vi "Abort-lasing.vi"(8 "error in (no error)":errorcluster, 11 "Object ref in":T1) -> (0 "error out":errorcluster, 3 "Object ref out":T1)   [LabVIEW 2013, in "SLMControl.lvlib" / "SC-Main.lvclass"]
uses:
  SC-Main.lvclass
  Object-reference.ctl
  UI/Control-names.ctl
  Vision-actions.ctl
  SC-Main.lvclass/SC-Main.ctl
  Read Lasing control.vi
  Read UI.vi
  UI/Set-control-boolean.vi
  UI/Set-control-string.vi
  SM1000/SM1000.lvclass
  UI/SC-UI.lvclass
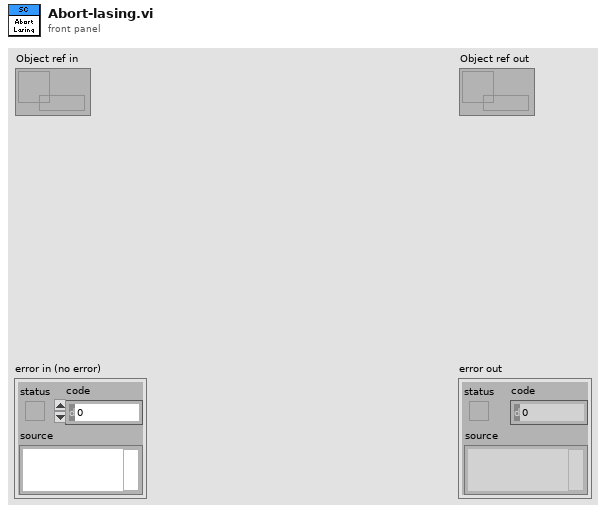
[diagram p1: front panel]
types:
  T1 = typedef "SLMControl.lvlib/SC-Main.lvclass/Object-reference.ctl" = refnum<data-value>
  T2 = typedef "SLMControl.lvlib/SC-Main.lvclass/Vision-actions.ctl" = enum16{"Activate", "Start", "Repeat", "Stop", "Exit"}
  T3 = typedef "SLMControl.lvlib/SC-UI.lvclass/Control-names.ctl" = enum16{"Com-in", "Com-out", "Help", "Status", "Load configuration", "Save configuration", "Load lasing files", "Load deposition files", "Clear", "Files", "Activate", "Execute", "Abort", "Options", "Current layer", "Current iteration", "Last elapsed time", "Deposition status", "Lasing job", "Status LEDs", "Exiting led", "Initialized led", "Files loaded led", "Activated led", "Executing led", "Deposition led", "Lasing job led", "Lasing led"}
  T4 = typedef "SLMControl.lvlib/SM1000.lvclass/Object-reference.ctl" = refnum<data-value>
  T5 = typedef "SLMControl.lvlib/SC-UI.lvclass/Panes-reference.ctl" = refnum<data-value>
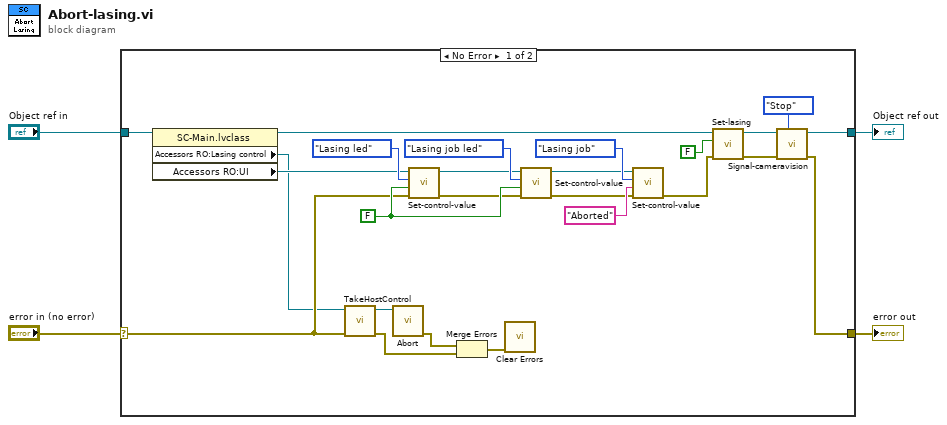
[diagram p0: block diagram]
diagram:
  n1 = case shown="No Error" "error in (no error)" {
    selector: "error in (no error)" -> [w13 w31]
    tunnel: [w7 w31] -> w3
    tunnel: [w5 w30] -> w1
    tunnel: "Object ref in" -> [w29 w30]
    frame No Error {
      w23 = FALSE
      n2 = property class="SC-Main.lvclass"(reference=w29) -> (reference out=w16:T1, "Accessors RO:Lasing control"=w11:T4, "Accessors RO:UI"=w17:T5)  [unwired: 1 in, 1 out]
      n3 = call "TakeHostControl.vi"("error in (no error)"=w13, "SM1000-control in"=w11) -> ("error out"=w12:errorcluster, "SM1000-control out"=w14:T4)  [unwired: 8 in]
      n4 = call "Abort.vi"("SM1000-control in"=w14) -> ("error out"=w15:errorcluster)  [unwired: 9 in, 1 out]
      n5 = call-poly "Set-control-value.vi"("error in (no error)"=w13, "Value"=w23, "Control name"=Control-names."Lasing led", "Panes in"=w17) -> ("error out"=w21:errorcluster, "Panes out"=w25:T5)  [unwired: 6 in]
      n6 = Merge Errors(w15, w12) -> (w10:errorcluster)
      n7 = call <vilib>:"Clear Errors.vi"("error in (no error)"=w10) -> ()  [unwired: 6 in, 1 out]
      n8 = call-poly "Set-control-value.vi"("error in (no error)"=w21, "Value"=w23, "Control name"=Control-names."Lasing job led", "Panes in"=w25) -> ("error out"=w20:errorcluster, "Panes out"=w24:T5)  [unwired: 6 in]
      n9 = call-poly "Set-control-value.vi"("error in (no error)"=w20, "Value"="Aborted", "Control name"=Control-names."Lasing job", "Panes in"=w24) -> ("error out"=w19:errorcluster)  [unwired: 6 in, 1 out]
      n10 = call "Set-lasing.vi"("error in (no error)"=w19, "Lasing?"=FALSE, "Object ref in"=w16) -> ("error out"=w8:errorcluster, "Object ref out"=w6:T1)  [unwired: 7 in]
      n11 = call "Signal-cameravision.vi"("Vision action"=Vision-actions."Stop", "error in (no error)"=w8, "Object ref in"=w6) -> ("error out"=w7:errorcluster, "Object ref out"=w5:T1)  [unwired: 7 in]
    }
    frame Error {
    }
  }
  "error out" <- w3
  "Object ref out" <- w1
